vi "Stop Steering Frame.vi"(8 "Steering Frame in":T3) -> (0 "Steering Frame out":T3)   [LabVIEW 2012]
uses:
  <vilib>/robotics/Steering/Class Type Definitions/Mecanum Steering Frame.ctl
  <vilib>/robotics/Steering/Mecanum Steering Frame/NI_Robotics_Mecanum Steering Frame.lvclass
  <vilib>/robotics/Steering/Class Type Definitions/Differential Steering Frame.ctl
  <vilib>/robotics/Steering/Differential Steering Frame/NI_Robotics_Differential Steering Frame.lvclass
  <vilib>/robotics/Steering/Steering Frame/Apply Steering Frame Velocity to Wheels.vi
  <vilib>/robotics/Steering/Steering Frame/NI_Robotics_Steering Frame.lvclass
  <vilib>/robotics/Steering/Class Type Definitions/NI_Robotics_Steering Class Types.lvlib
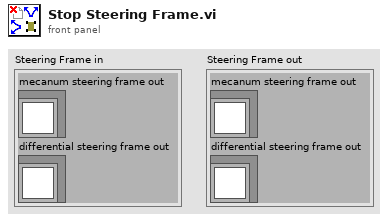
[diagram p1: front panel]
types:
  T1 = typedef "NI_Robotics_Steering Class Types.lvlib/Mecanum Steering Frame.ctl" = refnum<class "NI_Robotics_Mecanum Steering Frame.lvclass">
  T2 = typedef "NI_Robotics_Steering Class Types.lvlib/Differential Steering Frame.ctl" = refnum<class "NI_Robotics_Differential Steering Frame.lvclass">
  T3 = cluster{"mecanum steering frame out":T1, "differential steering frame out":T2}
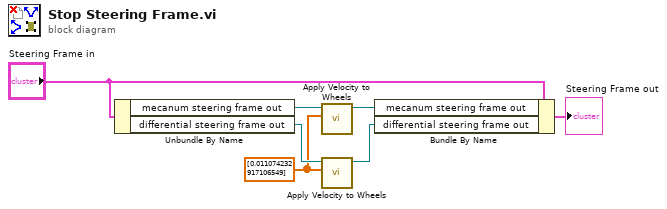
[diagram p0: block diagram]
diagram:
  w3 = dbl[] [0.011074232917106549] ("Channels out")
  n1 = Unbundle By Name("Steering Frame in") -> ("mecanum steering frame out"=w6:T1, "differential steering frame out"=w7:T2)
  n2 = call-poly <vilib>:"Apply Velocity to Wheels.vi"("steering frame velocity"=w3, "steering frame in"=w6) -> ("steering frame out"=w5:T1)  [unwired: 6 in, 3 out]
  n3 = call-poly <vilib>:"Apply Velocity to Wheels.vi"("steering frame velocity"=w3, "steering frame in"=w7) -> ("steering frame out"=w4:T2)  [unwired: 6 in, 3 out]
  n4 = Bundle By Name(cluster="Steering Frame in", "mecanum steering frame out"=w5, "differential steering frame out"=w4) -> (→"Steering Frame out":T3)
